vi "Disabled.vi"(7 "Robot Mode":T2, 10 "Match Info":T1={"Autonomous Elapsed Seconds"=0.0, "TeleOp Elapsed Seconds"=0.0, "Disabled Elapsed Seconds"=0.0, "Visited Autonomous"=FALSE, "Visited TeleOp"=FALSE, "Visited Disabled"=FALSE, "Autonomous Settings"={"Autonomous Style"=enum."Independent", "VI Refnum"=refnum}}, 11 "Call Context":T3) -> ()   [LabVIEW 2012]
doc: "This VI is called each time a disabled packet is received from the DS. It is often used to prepare for the next robot mode, to calibrate sensors, etc."
uses:
  <vilib>/Rock Robotics/WPI/DriverStation/WPI_DriverStationDerivedRobotMode.ctl
  <vilib>/Rock Robotics/WPI/DriverStation/WPI_DriverStationRobotMode2.ctl
  <vilib>/Rock Robotics/WPI/DriverStation/WPI_DriverStationMatch Info.ctl
  Robot Global Data.vi
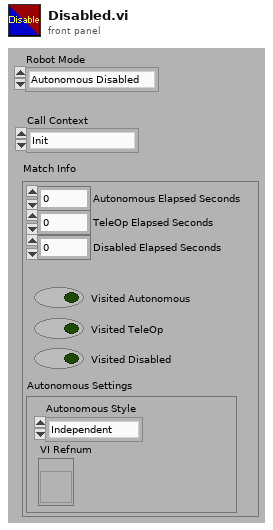
[diagram p1: front panel]
types:
  T1 = typedef "WPI_DriverStationMatch Info.ctl" = cluster{"Autonomous Elapsed Seconds":dbl, "TeleOp Elapsed Seconds":dbl, "Disabled Elapsed Seconds":dbl, "Visited Autonomous":bool, "Visited TeleOp":bool, "Visited Disabled":bool, "Autonomous Settings":cluster{"Autonomous Style":enum16{"Iterative", "Independent"}, "VI Refnum":refnum<vi>}}
  T2 = typedef "WPI_DriverStationRobotMode2.ctl" = enum16{"Autonomous Disabled", "Autonomous Enabled", "Teleop Disabled", "Teleop Enabled", "Timeout", "Finish", "Test Disabled", "Test Enabled"}
  T3 = typedef "WPI_DriverStationDerivedRobotMode.ctl" = enum16{"Init", "Execute", "Stop"}
  T4 = typedef "WPI_MotorControlDeviceRef.ctl" = cluster{"DeviceStatus":errorcluster, "Type":enum16{"PWM", "CAN"}, "PWM":cluster{"Digital Module":T5, "PWM Channel":T6, "DeadBand":T7}, "CAN":cluster{"Device Number":u8, "Control Mode":T8, "Semaphore":T9, "Max Vout":dbl}, "Invert":bool, "TransformRef":T10, "InvTransformRef":T10}
  T5 = typedef "FPGA_TypedefDigitalModule.ctl" = enum16{"Digital Module 1", "Digital Module 2"}
  T6 = typedef "FPGA_DIOPWMChannel.ctl" = enum8{"PWM 1", "PWM 2", "PWM 3", "PWM 4", "PWM 5", "PWM 6", "PWM 7", "PWM 8", "PWM 9", "PWM 10", "Invalid"}
  T7 = typedef "WPI_PWMDeadband.ctl" = cluster{"Name":string, "maxPositivePwm":i32, "minPositivePwm":i32, "centerPwm":i32, "maxNegativePwm":i32, "minNegativePwm":i32, "angularRange":u16}
  T8 = typedef "WPI_CANJaguar_ControlMode.ctl" = enum8{"Percent VBus", "Current", "Speed", "Position", "Voltage"}
  T9 = typedef "Semaphore RefNum" = refnum<k1>
  T10 = typedef "WPI_PWMTransform_ConPane.ctl" = refnum<vi>
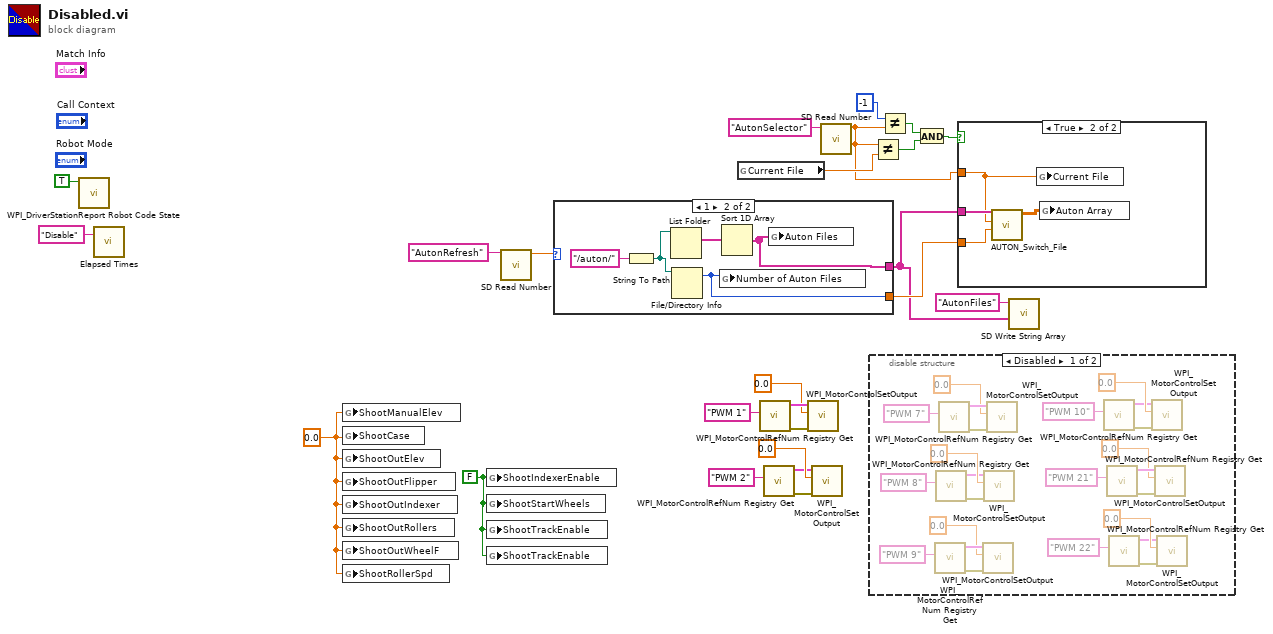
[diagram p0: block diagram]
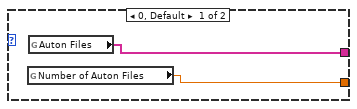
[diagram p4: hidden frame]
diagram:
  w22 = FALSE ("ShootIndexerEnable")
  w21 = 0.0 ("ShootCase")
  n1 = call <vilib>:"WPI_DriverStationReport Robot Code State.vi"("Disabled"=TRUE ("Autonomous")) -> ()  [unwired: 10 in, 1 out]
  n2 = call "Elapsed Times.vi"("Call Name"="Disable") -> ()  [unwired: 2 in, 1 out]
  n3 = global write "Robot Global Data.vi" "ShootManualElev"(w21) -> ()
  n4 = global write "Robot Global Data.vi" "ShootCase"(w21) -> ()
  n5 = global write "Robot Global Data.vi" "ShootOutElev"(w21) -> ()
  n6 = global write "Robot Global Data.vi" "ShootOutFlipper"(w21) -> ()
  n7 = global write "Robot Global Data.vi" "ShootOutIndexer"(w21) -> ()
  n8 = global write "Robot Global Data.vi" "ShootOutRollers"(w21) -> ()
  n9 = global write "Robot Global Data.vi" "ShootOutWheelF"(w21) -> ()
  n10 = global write "Robot Global Data.vi" "ShootRollerSpd"(w21) -> ()
  n11 = global write "Robot Global Data.vi" "ShootIndexerEnable"(w22) -> ()
  n12 = global write "Robot Global Data.vi" "ShootStartWheels"(w22) -> ()
  n13 = global write "Robot Global Data.vi" "ShootTrackEnable"(w22) -> ()
  n14 = global write "Robot Global Data.vi" "ShootTrackEnable"(w22) -> ()
  n15 = call <vilib>:"SD Read Number.vi"("Name"="AutonRefresh") -> ("Numeric"=w2:dbl)  [unwired: 8 in, 2 out]
  n16 = case shown="1" w2 {
    tunnel: [w25 w28] -> w12
    tunnel: [w26 w27] -> w7
    frame 0, Default {
      n17 = global read "Robot Global Data.vi" "Number of Auton Files"() -> (w25:dbl)
      n18 = global read "Robot Global Data.vi" "Auton Files"() -> (w26:string[])
    }
    frame 1 {
      n19 = String To Path(string="/auton/") -> (path=w30:path)
      n20 = List Folder(path=w30) -> (filenames=w29:string[])  [unwired: 3 in, 3 out]
      n21 = File/Directory Info(path=w30) -> (size=w28:i64)  [unwired: 1 in, 6 out]
      n22 = global write "Robot Global Data.vi" "Number of Auton Files"(w28) -> ()
      n23 = Sort 1D Array(array=w29) -> (sorted array=w27:string[])
      n24 = global write "Robot Global Data.vi" "Auton Files"(w27) -> ()
    }
  }
  n25 = global read "Robot Global Data.vi" "Current File"() -> (w10:dbl)
  n26 = call <vilib>:"WPI_MotorControlRefNum Registry Get.vi"("refnum name"="PWM 1") -> ("error out"=w20:errorcluster, "MotorControlDevRef"=w19:T4)  [unwired: 9 in]
  n27 = call <vilib>:"WPI_MotorControlRefNum Registry Get.vi"("refnum name"="PWM 2") -> ("error out"=w13:errorcluster, "MotorControlDevRef"=w14:T4)  [unwired: 9 in]
  n28 = call <vilib>:"WPI_MotorControlSetOutput.vi"("error in (no error)"=w20, "Output"=0.0, "MotorControlDevRef"=w19) -> ()  [unwired: 6 in, 3 out]
  n29 = call <vilib>:"WPI_MotorControlSetOutput.vi"("error in (no error)"=w13, "Output"=0.0, "MotorControlDevRef"=w14) -> ()  [unwired: 6 in, 3 out]
  n30 = call <vilib>:"SD Read Number.vi"("Name"="AutonSelector") -> ("Numeric"=w3:dbl)  [unwired: 8 in, 2 out]
  n31 = disable-structure shown="Disabled" {
    frame Disabled {
      n32 = call <vilib>:"WPI_MotorControlRefNum Registry Get.vi"("refnum name"="PWM 9") -> ("error out"=w47:errorcluster, "MotorControlDevRef"=w46:T4)  [unwired: 9 in]
      n33 = call <vilib>:"WPI_MotorControlRefNum Registry Get.vi"("refnum name"="PWM 8") -> ("error out"=w48:errorcluster, "MotorControlDevRef"=w49:T4)  [unwired: 9 in]
      n34 = call <vilib>:"WPI_MotorControlRefNum Registry Get.vi"("refnum name"="PWM 7") -> ("error out"=w55:errorcluster, "MotorControlDevRef"=w54:T4)  [unwired: 9 in]
      n35 = call <vilib>:"WPI_MotorControlSetOutput.vi"("error in (no error)"=w47, "Output"=0.0, "MotorControlDevRef"=w46) -> ()  [unwired: 6 in, 3 out]
      n36 = call <vilib>:"WPI_MotorControlSetOutput.vi"("error in (no error)"=w48, "Output"=0.0, "MotorControlDevRef"=w49) -> ()  [unwired: 6 in, 3 out]
      n37 = call <vilib>:"WPI_MotorControlSetOutput.vi"("error in (no error)"=w55, "Output"=0.0, "MotorControlDevRef"=w54) -> ()  [unwired: 6 in, 3 out]
      n38 = call <vilib>:"WPI_MotorControlRefNum Registry Get.vi"("refnum name"="PWM 10") -> ("error out"=w40:errorcluster, "MotorControlDevRef"=w41:T4)  [unwired: 9 in]
      n39 = call <vilib>:"WPI_MotorControlRefNum Registry Get.vi"("refnum name"="PWM 21") -> ("error out"=w39:errorcluster, "MotorControlDevRef"=w38:T4)  [unwired: 9 in]
      n40 = call <vilib>:"WPI_MotorControlRefNum Registry Get.vi"("refnum name"="PWM 22") -> ("error out"=w32:errorcluster, "MotorControlDevRef"=w33:T4)  [unwired: 9 in]
      n41 = call <vilib>:"WPI_MotorControlSetOutput.vi"("error in (no error)"=w40, "Output"=0.0, "MotorControlDevRef"=w41) -> ()  [unwired: 6 in, 3 out]
      n42 = call <vilib>:"WPI_MotorControlSetOutput.vi"("error in (no error)"=w39, "Output"=0.0, "MotorControlDevRef"=w38) -> ()  [unwired: 6 in, 3 out]
      n43 = call <vilib>:"WPI_MotorControlSetOutput.vi"("error in (no error)"=w32, "Output"=0.0, "MotorControlDevRef"=w33) -> ()  [unwired: 6 in, 3 out]
    }
    frame Enabled {
    }
  }
  n44 = Not Equal?(x=w3, y=w10) -> (x != y?=w8:bool)
  n45 = Not Equal?(x=-1, y=w3) -> (x != y?=w9:bool)
  n46 = And(x=w9, y=w8) -> (x .and. y?=w5:bool)
  n47 = case shown="True" w5 {
    tunnel: w7 -> [_ w59]
    tunnel: w12 -> [_ w58]
    tunnel: w3 -> [_ w56]
    frame False {
    }
    frame True {
      n48 = call "AUTON_Switch_File.vi"("Number of Auton Files"=w58, "Auton File"=w56, "Auton Files"=w59) -> ("Auton Array"=w57:dbl[][])  [unwired: 7 in, 1 out]
      n49 = global write "Robot Global Data.vi" "Current File"(w56) -> ()
      n50 = global write "Robot Global Data.vi" "Auton Array"(w57) -> ()
    }
  }
  n51 = call <vilib>:"SD Write String Array.vi"("String Array"=w7, "Name"="AutonFiles") -> ()  [unwired: 8 in, 2 out]
